vi "Lift Action.vi"(8 "Motor Safety":T1, 11 "Operation States":T3) -> ()   [LabVIEW 2014]
uses:
  <vilib>/Rock Robotics/WPI/SafetyOutput/WPI_SafetyOutputConfigMenu.ctl
  <vilib>/Rock Robotics/WPI/Solenoid/WPI_SolenoidValue.ctl
  <vilib>/Rock Robotics/WPI/Solenoid/WPI_SolenoidSetEnum.vi
  Robot Global Data.vi
panel:
  in  "Motor Safety":T1
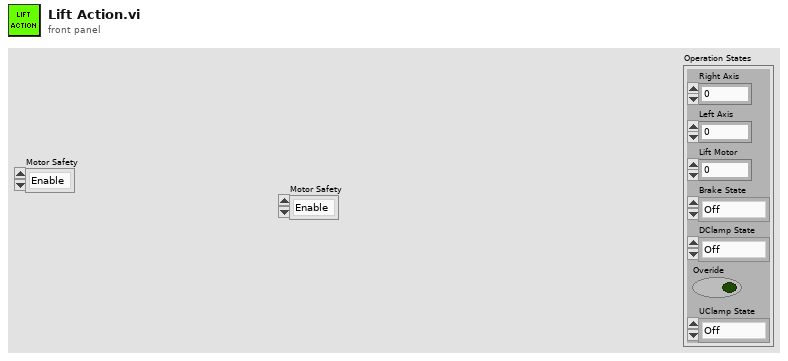
[diagram p1: front panel]
types:
  T1 = typedef "WPI_SafetyOutputConfigMenu.ctl" = enum16{"Enable", "Disable"}
  T2 = typedef "WPI_SolenoidValue.ctl" = enum16{"Off", "On", "Forward", "Reverse"}
  T3 = cluster{"Right Axis":dbl, "Left Axis":dbl, "Lift Motor":dbl, "Brake State":T2, "DClamp State":T2, "Overide":bool, "UClamp State":T2}
  T4 = typedef "WPI_SolenoidDevRef.ctl" = cluster{"DevStatus":errorcluster, "Pneumatics Control Module":u8, "Forward Solenoid Channel":T5, "Reverse Solenoid Channel":T5}
  T5 = typedef "WPI_SolenoidChannel.ctl" = enum8{"Solenoid 0", "Solenoid 1", "Solenoid 2", "Solenoid 3", "Solenoid 4", "Solenoid 5", "Solenoid 6", "Solenoid 7", "Invalid"}
  T6 = typedef "WPI_MotorControlDeviceRef.ctl" = cluster{"DeviceStatus":errorcluster, "Type":T7, "PWM":cluster{"Controller":T8, "PWM Channel":T9, "DeadBand":T10}, "CAN":cluster{"Device Number":u8, "Control Mode":T11, "Semaphore":T12, "Max Vout":dbl, "TalonSRX Control Mode":T13}, "Invert":bool, "TransformRef":T14, "InvTransformRef":T14}
  T7 = typedef "WPI_MotorControlType.ctl" = enum16{"PWM", "CAN", "CANTalonSRX"}
  T8 = typedef "FPGA_TypedefDigitalModule.ctl" = enum16{"Controller 1"}
  T9 = typedef "FPGA_DIOPWMChannel.ctl" = enum8{"PWM 0", "PWM 1", "PWM 2", "PWM 3", "PWM 4", "PWM 5", "PWM 6", "PWM 7", "PWM 8", "PWM 9", "PWM MXP 0", "PWM MXP 1", "PWM MXP 2", "PWM MXP 3", "PWM MXP 4", "PWM MXP 5", "PWM MXP 6", "PWM MXP 7", "PWM MXP 8", "PWM MXP 9", "Invalid"}
  T10 = typedef "WPI_PWMDeadband.ctl" = cluster{"Name":string, "maxPositivePwm":i32, "minPositivePwm":i32, "centerPwm":i32, "maxNegativePwm":i32, "minNegativePwm":i32, "angularRange":u16}
  T11 = typedef "WPI_CANJaguar_ControlMode.ctl" = enum8{"Percent VBus", "Current", "Speed", "Position", "Voltage"}
  T12 = typedef "Semaphore RefNum" = refnum<k1>
  T13 = typedef "WPI_CANTalonSRX_APIControlMode.ctl" = enum8{"Percent VBus", "Speed", "Position", "Slave", "Unchanged / Invalid"}
  T14 = typedef "WPI_PWMTransform_ConPane.ctl" = refnum<vi>
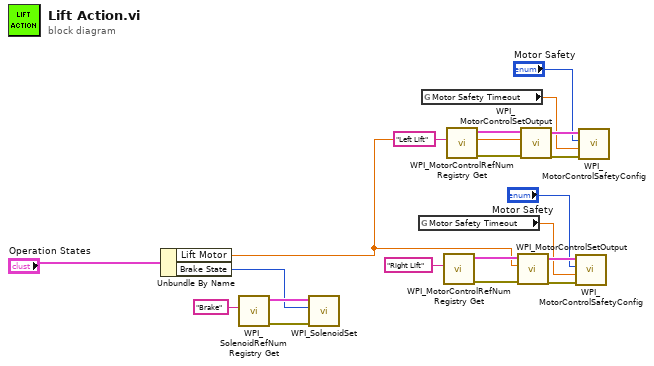
[diagram p0: block diagram]
diagram:
  n1 = Unbundle By Name("Operation States") -> ("Lift Motor"=w1:dbl, "Brake State"=w10:T2)
  n2 = call <vilib>:"WPI_SolenoidRefNum Registry Get.vi"("refnum name"="Brake") -> ("error out"=w12:errorcluster, "SolenoidDevRef"=w11:T4)  [unwired: 9 in]
  n3 = call-poly <vilib>:"WPI_SolenoidSet.vi"("error in (no error)"=w12, "Value"=w10, "SolenoidDevRef"=w11) -> ()  [unwired: 7 in, 2 out]
  n4 = global read "Robot Global Data.vi" "Motor Safety Timeout"() -> (w2:dbl)
  n5 = global read "Robot Global Data.vi" "Motor Safety Timeout"() -> (w14:dbl)
  n6 = call <vilib>:"WPI_MotorControlRefNum Registry Get.vi"("refnum name"="Right Lift") -> ("error out"=w7:errorcluster, "MotorControlDevRef"=w6:T6)  [unwired: 9 in]
  n7 = call <vilib>:"WPI_MotorControlRefNum Registry Get.vi"("refnum name"="Left Lift") -> ("error out"=w19:errorcluster, "MotorControlDevRef"=w18:T6)  [unwired: 9 in]
  n8 = call <vilib>:"WPI_MotorControlSetOutput.vi"("error in (no error)"=w7, "Output"=w1, "MotorControlDevRef"=w6) -> ("error out"=w5:errorcluster, "MotorControlDevRef"=w4:T6)  [unwired: 6 in, 1 out]
  n9 = call <vilib>:"WPI_MotorControlSetOutput.vi"("error in (no error)"=w19, "Output"=w1, "MotorControlDevRef"=w18) -> ("error out"=w17:errorcluster, "MotorControlDevRef"=w16:T6)  [unwired: 6 in, 1 out]
  n10 = call <vilib>:"WPI_MotorControlSafetyConfig.vi"("error in (no error)"=w5, "timeout (s)"=w2, "mode"="Motor Safety", "MotorControlDevRef"=w4) -> ()  [unwired: 6 in, 2 out]
  n11 = call <vilib>:"WPI_MotorControlSafetyConfig.vi"("error in (no error)"=w17, "timeout (s)"=w14, "mode"="Motor Safety", "MotorControlDevRef"=w16) -> ()  [unwired: 6 in, 2 out]
